vi "Variable_12kW.vi"() -> ()   [LabVIEW 2020]
panel:
  out "Voltage (V)":dbl
  in  "Power Supply":bool
  out "B":bool
  out "Y":bool
  out "R":bool
  out "No. of Resistors Used":i32
  in  "Step Type":enum32{"Variable Steps", "Equal Steps"}(tab)
  out "Step 7\nIndicator":bool
  out "Step 4\nIndicator":bool
  out "Step 10\nIndicator":bool
  out "Step 9\nIndicator":bool
  out "Step 8\nIndicator":bool
  out "Step 6\nIndicator":bool
  out "Step 5\nIndicator":bool
  out "Step 3\nIndicator":bool
  out "Step 2\nIndicator":bool
  out "Step 1\nIndicator":bool
  in  "Step 1\n250W":bool
  in  "Step 2\n250W":bool
  in  "Step 3\n500W":bool
  in  "Step 4\n1000W":bool
  in  "Step 5\n1000W":bool
  in  "Step 6\n1000W":bool
  in  "Step 7\n2000W":bool
  in  "Step 8\n2000W":bool
  in  "Step 9\n2000W":bool
  in  "Step 10\n2000W":bool
  in  "No. of Equal Steps":T1(tab)
  in  "Step 2\n6000W":bool
  in  "Step 1\n6000W":bool
  out "Step 1\nIndicator 3":bool
  out "Step 2\nIndicator 3":bool
  in  "Step 3\n4000W":bool
  in  "Step 2\n4000W":bool
  in  "Step 1\n4000W":bool
  out "Step 1\nIndicator 4":bool
  out "Step 2\nIndicator 4":bool
  out "Step 3\nIndicator 3":bool
  in  "Step 4\n3000W":bool
  in  "Step 3\n3000W":bool
  in  "Step 2\n3000W":bool
  in  "Step 1\n3000W":bool
  out "Step 1\nIndicator 5":bool
  out "Step 2\nIndicator 5":bool
  out "Step 3\nIndicator 4":bool
  out "Step 4\nIndicator 3":bool
  in  "Step 6\n2000W":bool
  in  "Step 5\n2000W":bool
  in  "Step 4\n2000W":bool
  in  "Step 3\n2000W":bool
  in  "Step 2\n2000W":bool
  in  "Step 1\n2000W":bool
  out "Step 1\nIndicator 2":bool
  out "Step 2\nIndicator 2":bool
  out "Step 3\nIndicator 2":bool
  out "Step 5\nIndicator 2":bool
  out "Step 6\nIndicator 2":bool
  out "Step 4\nIndicator 2":bool
  in  "Master Switch":bool
  out "Load (kW)":dbl
  out "Current (A)":dbl format="%.4f"
  # "Three Phase Variable Resistive Load Bank with 12kW Maximum Capacity and 10 Step Control"
  # "All resistors are connected in 3 phase star formation"
  # "3 Phase Voltage Indicator"
  # "Resistors in Use"
  # "Resistors in Use"
  # "Resistors in Use"
  # "Resistors in Use"
  # "Resistors in Use"
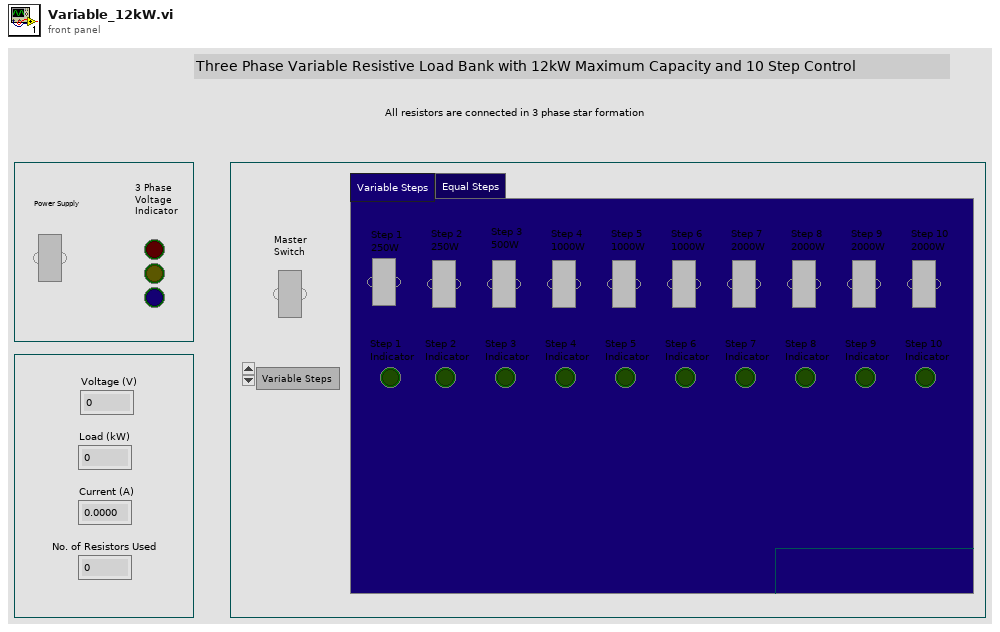
[diagram p1: front panel]
types:
  T1 = enum32{"2 Steps", "3 Steps", "4 Steps", "6 Steps"}
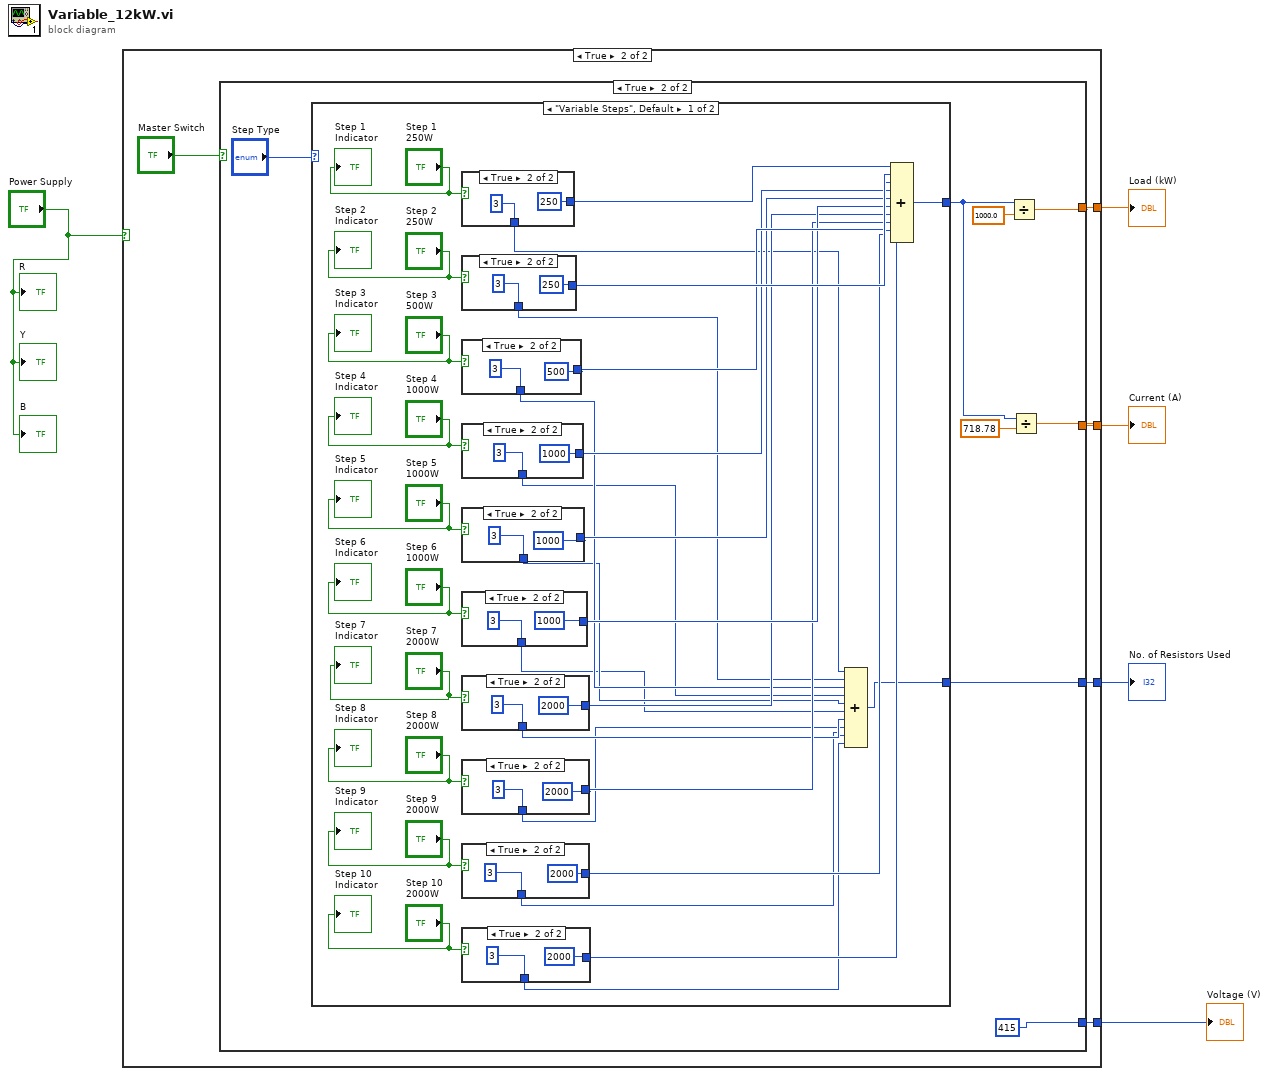
[diagram p0: block diagram]
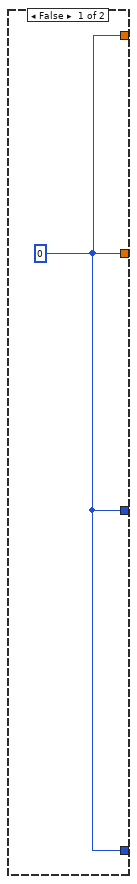
[diagram p2: hidden frame]
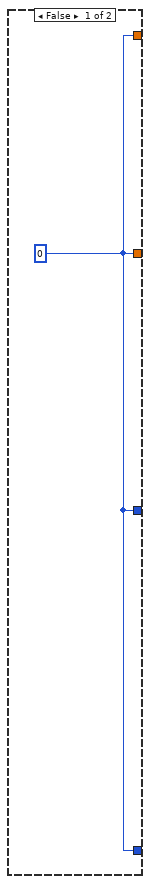
[diagram p3: hidden frame]
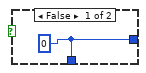
[diagram p4: hidden frame]
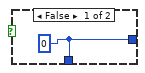
[diagram p5: hidden frame]
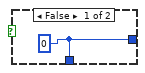
[diagram p6: hidden frame]
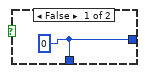
[diagram p7: hidden frame]
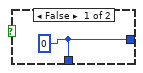
[diagram p8: hidden frame]
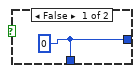
[diagram p9: hidden frame]
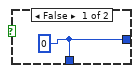
[diagram p10: hidden frame]
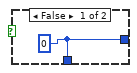
[diagram p11: hidden frame]
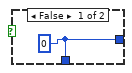
[diagram p12: hidden frame]
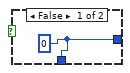
[diagram p13: hidden frame]
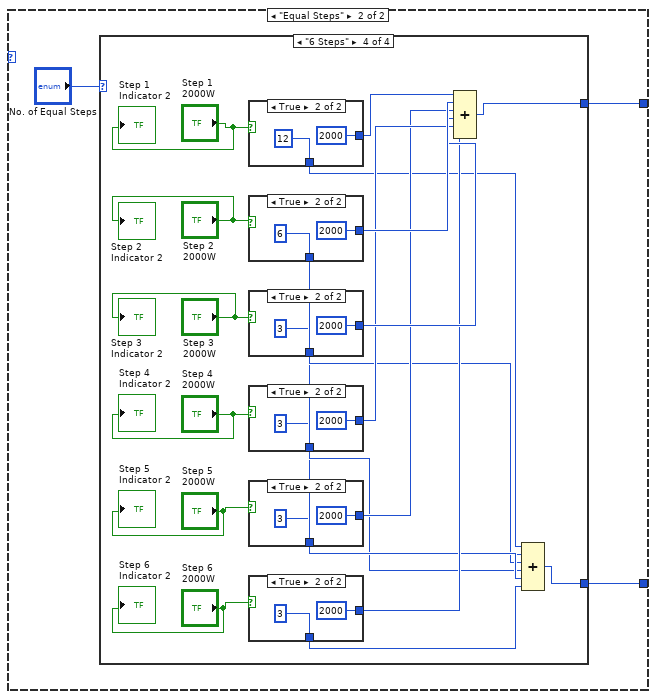
[diagram p14: hidden frame]
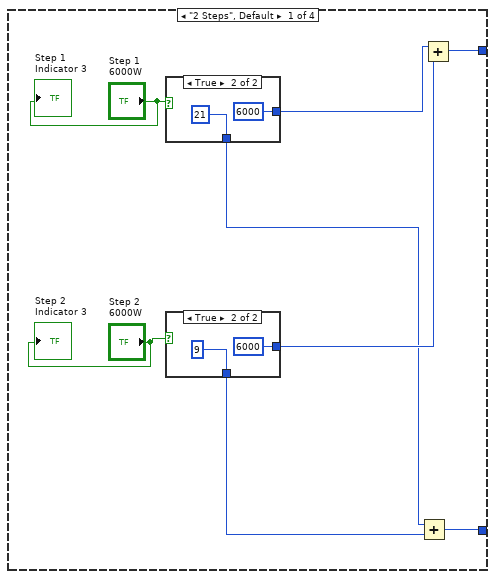
[diagram p15: hidden frame]
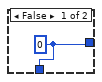
[diagram p16: hidden frame]
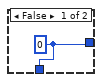
[diagram p17: hidden frame]
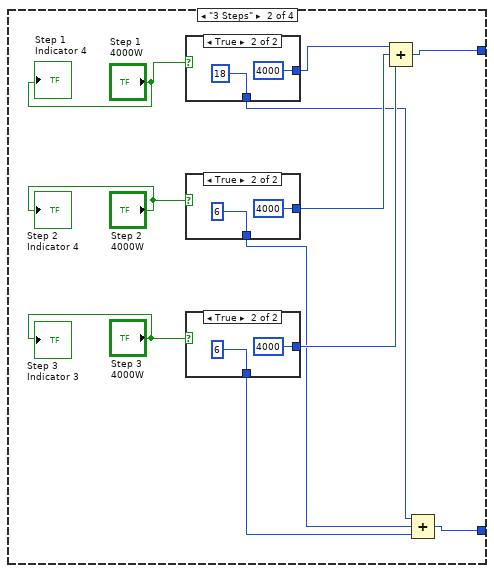
[diagram p18: hidden frame]
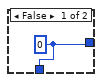
[diagram p19: hidden frame]
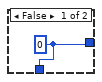
[diagram p20: hidden frame]
diagram:
  n1 = case shown="True" "Power Supply" {
    tunnel: [w6 w10] -> w5
    tunnel: [w6 w9] -> w3
    tunnel: [w6 w8] -> w4
    tunnel: [w6 w7] -> w1
    frame False {
      w6 = 0
    }
    frame True {
      n2 = case shown="True" "Master Switch" {
        tunnel: [w12 w20] -> w8
        tunnel: [w12 w14] -> w9
        tunnel: [w12 w16] -> w10
        tunnel: [w12 415] -> w7
        frame False {
          w12 = 0
        }
        frame True {
          n3 = case shown="\"Variable Steps\", Default" "Step Type" {
            tunnel: [w22 w83] -> w20
            tunnel: [w21 w84] -> w13
            frame "Variable Steps", Default {
              n4 = case shown="True" "Step 1\n250W" {
                tunnel: [w80 250] -> w42
                tunnel: [w80 3] -> w32
                frame False {
                  w80 = 0
                }
                frame True {
                }
              }
              n5 = case shown="True" "Step 2\n250W" {
                tunnel: [w77 250] -> w41
                tunnel: [w77 3] -> w31
                frame False {
                  w77 = 0
                }
                frame True {
                }
              }
              n6 = case shown="True" "Step 3\n500W" {
                tunnel: [w74 500] -> w40
                tunnel: [w74 3] -> w30
                frame False {
                  w74 = 0
                }
                frame True {
                }
              }
              n7 = case shown="True" "Step 4\n1000W" {
                tunnel: [w71 1000] -> w39
                tunnel: [w71 3] -> w29
                frame False {
                  w71 = 0
                }
                frame True {
                }
              }
              n8 = case shown="True" "Step 5\n1000W" {
                tunnel: [w68 1000] -> w38
                tunnel: [w68 3] -> w28
                frame False {
                  w68 = 0
                }
                frame True {
                }
              }
              n9 = case shown="True" "Step 6\n1000W" {
                tunnel: [w65 1000] -> w37
                tunnel: [w65 3] -> w27
                frame False {
                  w65 = 0
                }
                frame True {
                }
              }
              n10 = case shown="True" "Step 7\n2000W" {
                tunnel: [w62 2000] -> w36
                tunnel: [w62 3] -> w26
                frame False {
                  w62 = 0
                }
                frame True {
                }
              }
              n11 = case shown="True" "Step 8\n2000W" {
                tunnel: [w59 2000] -> w35
                tunnel: [w59 3] -> w25
                frame False {
                  w59 = 0
                }
                frame True {
                }
              }
              n12 = case shown="True" "Step 9\n2000W" {
                tunnel: [w56 2000] -> w34
                tunnel: [w56 3] -> w24
                frame False {
                  w56 = 0
                }
                frame True {
                }
              }
              n13 = case shown="True" "Step 10\n2000W" {
                tunnel: [w53 2000] -> w33
                tunnel: [w53 3] -> w23
                frame False {
                  w53 = 0
                }
                frame True {
                }
              }
              n14 = Compound Arithmetic op=ADD(w32, w31, w30, w29, w28, w27, w26, w25, w24, w23) -> (w22:i32)
              n15 = Compound Arithmetic op=ADD(w42, w41, w40, w39, w38, w37, w36, w35, w34, w33) -> (w21:i32)
              "Step 1\nIndicator" <- "Step 1\n250W"
              "Step 4\nIndicator" <- "Step 4\n1000W"
              "Step 7\nIndicator" <- "Step 7\n2000W"
              "Step 2\nIndicator" <- "Step 2\n250W"
              "Step 3\nIndicator" <- "Step 3\n500W"
              "Step 5\nIndicator" <- "Step 5\n1000W"
              "Step 8\nIndicator" <- "Step 8\n2000W"
              "Step 9\nIndicator" <- "Step 9\n2000W"
              "Step 10\nIndicator" <- "Step 10\n2000W"
              "Step 6\nIndicator" <- "Step 6\n1000W"
            }
            frame "Equal Steps" {
              n16 = case shown="\"6 Steps\"" "No. of Equal Steps" {
                tunnel: [w86 w107 w129 w159] -> w84
                tunnel: [w89 w100 w120 w152] -> w83
                frame "2 Steps", Default {
                  n17 = case shown="True" "Step 1\n6000W" {
                    tunnel: [w97 21] -> w88
                    tunnel: [w97 6000] -> w91
                    frame False {
                      w97 = 0
                    }
                    frame True {
                    }
                  }
                  n18 = case shown="True" "Step 2\n6000W" {
                    tunnel: [w94 9] -> w87
                    tunnel: [w94 6000] -> w90
                    frame False {
                      w94 = 0
                    }
                    frame True {
                    }
                  }
                  n19 = Add(x=w88, y=w87) -> (x+y=w89:i32)
                  n20 = Add(x=w91, y=w90) -> (x+y=w86:i32)
                  "Step 2\nIndicator 3" <- "Step 2\n6000W"
                  "Step 1\nIndicator 3" <- "Step 1\n6000W"
                }
                frame "3 Steps" {
                  n21 = case shown="True" "Step 1\n4000W" {
                    tunnel: [w117 18] -> w103
                    tunnel: [w117 4000] -> w106
                    frame False {
                      w117 = 0
                    }
                    frame True {
                    }
                  }
                  n22 = case shown="True" "Step 2\n4000W" {
                    tunnel: [w114 6] -> w102
                    tunnel: [w114 4000] -> w105
                    frame False {
                      w114 = 0
                    }
                    frame True {
                    }
                  }
                  n23 = case shown="True" "Step 3\n4000W" {
                    tunnel: [w111 6] -> w101
                    tunnel: [w111 4000] -> w104
                    frame False {
                      w111 = 0
                    }
                    frame True {
                    }
                  }
                  n24 = Compound Arithmetic op=ADD(w106, w105, w104) -> (w107:i32)
                  n25 = Compound Arithmetic op=ADD(w103, w102, w101) -> (w100:i32)
                  "Step 1\nIndicator 4" <- "Step 1\n4000W"
                  "Step 3\nIndicator 3" <- "Step 3\n4000W"
                  "Step 2\nIndicator 4" <- "Step 2\n4000W"
                }
                frame "4 Steps" {
                  n26 = case shown="True" "Step 1\n3000W" {
                    tunnel: [w143 12] -> w124
                    tunnel: [w143 3000] -> w128
                    frame False {
                      w143 = 0
                    }
                    frame True {
                    }
                  }
                  n27 = case shown="True" "Step 2\n3000W" {
                    tunnel: [w140 6] -> w123
                    tunnel: [w140 3000] -> w127
                    frame False {
                      w140 = 0
                    }
                    frame True {
                    }
                  }
                  n28 = case shown="True" "Step 3\n3000W" {
                    tunnel: [w137 6] -> w122
                    tunnel: [w137 3000] -> w126
                    frame False {
                      w137 = 0
                    }
                    frame True {
                    }
                  }
                  n29 = case shown="True" "Step 4\n3000W" {
                    tunnel: [w134 6] -> w121
                    tunnel: [w134 3000] -> w125
                    frame False {
                      w134 = 0
                    }
                    frame True {
                    }
                  }
                  n30 = Compound Arithmetic op=ADD(w128, w127, w126, w125) -> (w129:i32)
                  n31 = Compound Arithmetic op=ADD(w124, w123, w122, w121) -> (w120:i32)
                  "Step 3\nIndicator 4" <- "Step 3\n3000W"
                  "Step 2\nIndicator 5" <- "Step 2\n3000W"
                  "Step 1\nIndicator 5" <- "Step 1\n3000W"
                  "Step 4\nIndicator 3" <- "Step 4\n3000W"
                }
                frame "6 Steps" {
                  n32 = case shown="True" "Step 1\n2000W" {
                    tunnel: [w181 12] -> w146
                    tunnel: [w181 2000] -> w158
                    frame False {
                      w181 = 0
                    }
                    frame True {
                    }
                  }
                  n33 = case shown="True" "Step 2\n2000W" {
                    tunnel: [w178 6] -> w147
                    tunnel: [w178 2000] -> w157
                    frame False {
                      w178 = 0
                    }
                    frame True {
                    }
                  }
                  n34 = case shown="True" "Step 3\n2000W" {
                    tunnel: [w175 3] -> w148
                    tunnel: [w175 2000] -> w156
                    frame False {
                      w175 = 0
                    }
                    frame True {
                    }
                  }
                  n35 = case shown="True" "Step 4\n2000W" {
                    tunnel: [w172 3] -> w149
                    tunnel: [w172 2000] -> w155
                    frame False {
                      w172 = 0
                    }
                    frame True {
                    }
                  }
                  n36 = case shown="True" "Step 5\n2000W" {
                    tunnel: [w169 3] -> w150
                    tunnel: [w169 2000] -> w154
                    frame False {
                      w169 = 0
                    }
                    frame True {
                    }
                  }
                  n37 = case shown="True" "Step 6\n2000W" {
                    tunnel: [w166 3] -> w151
                    tunnel: [w166 2000] -> w153
                    frame False {
                      w166 = 0
                    }
                    frame True {
                    }
                  }
                  n38 = Compound Arithmetic op=ADD(w158, w157, w154, w156, w155, w153) -> (w159:i32)
                  n39 = Compound Arithmetic op=ADD(w146, w147, w148, w149, w150, w151) -> (w152:i32)
                  "Step 1\nIndicator 2" <- "Step 1\n2000W"
                  "Step 6\nIndicator 2" <- "Step 6\n2000W"
                  "Step 5\nIndicator 2" <- "Step 5\n2000W"
                  "Step 2\nIndicator 2" <- "Step 2\n2000W"
                  "Step 3\nIndicator 2" <- "Step 3\n2000W"
                  "Step 4\nIndicator 2" <- "Step 4\n2000W"
                }
              }
            }
          }
          n40 = Divide(x=w13, y=1000.0) -> (x/y=w16:dbl)
          n41 = Divide(x=w13, y=718.78) -> (x/y=w14:dbl)
        }
      }
    }
  }
  "Load (kW)" <- w5
  "Current (A)" <- w3
  "No. of Resistors Used" <- w4
  "Voltage (V)" <- w1
  "B" <- "Power Supply"
  "Y" <- "Power Supply"
  "R" <- "Power Supply"
